vi "Get_Stat_Dots&Single_Frame_Displ-4.vi"(7 "Closing gaps":i32 min=1, 8 "[IN] error":errorcluster, 9 "[IN] Movie Values":T2 {"Particle Fil Setups"."Type of particle filter"."Measurement Parameter" items=["Center of Mass X", "Center of Mass Y", "First Pixel X", "First Pixel Y", "Bounding Rect Left", "Bounding Rect Top", "Bounding Rect Right", "Bounding Rect Bottom", "Max Feret Diameter Start X", "Max Feret Diameter Start Y", "Max Feret Diameter End X", "Max Feret Diameter End Y", "Max Horiz. Segment Length Left", "Max Horiz. Segment Length Right", "Max Horiz. Segment Length Row", "-", "Bounding Rect Width", "Bounding Rect Height", "Bounding Rect Diagonal", "Perimeter", "Convex Hull Perimeter", "Holes' Perimeter", "Max Feret Diameter", "Equivalent Ellipse Major Axis", "Equivalent Ellipse Minor Axis", "Equivalent Ellipse Minor Axis (Feret)", "Equivalent Rect Long Side", "Equivalent Rect Short Side", "Equivalent Rect Diagonal", "Equivalent Rect Short Side (Feret)", "Average Horiz. Segment Length", "Average Vert. Segment Length", "Hydraulic Radius", "Waddel Disk Diameter", "-", "Area", "Holes' Area", "Particle & Holes' Area", "Convex Hull Area", "Image Area", "-", "Number of Holes", "Number of Horiz. Segments", "Number of Vert. Segments", "-", "Orientation", "Max Feret Diameter Orientation", "-", "% Area/Image Area", "% Area/(Particle & Holes' Area)", "Ratio of Equivalent Ellipse Axes", "Ratio of Equivalent Rect Sides", "-", "Elongation Factor", "Compactness Factor", "Heywood Circularity Factor", "Type Factor", "-", "Sum X", "Sum Y", "Sum XX", "Sum XY", "Sum YY", "Sum XXX", "Sum XXY", "Sum XYY", "Sum YYY", "-", "Moment of Inertia XX", "Moment of Inertia XY", "Moment of Inertia YY", "Moment of Inertia XXX", "Moment of Inertia XXY", "Moment of Inertia XYY", "Moment of Inertia YYY", "Norm. Moment of Inertia XX", "Norm. Moment of Inertia XY", "Norm. Moment of Inertia YY", "Norm. Moment of Inertia XXX", "Norm. Moment of Inertia XXY", "Norm. Moment of Inertia XYY", "Norm. Moment of Inertia YYY", "Hu Moment 1", "Hu Moment 2", "Hu Moment 3", "Hu Moment 4", "Hu Moment 5", "Hu Moment 6", "Hu Moment 7"]}, 10 "dR max":dbl, 11 "dR min":dbl) -> (0 "error OUT":errorcluster, 1 "[OUT] Stationary Dots":T3(array[cluster]), 2 "[OUT] Displacements \nwith Length >1 Frame":dbl[][](array[numeric]), 3 "[OUT] (X,Y) Poten-\ntially Moving":dbl[][](array[numeric]), 5 "[OUT] Dot matrix after using \nsome filters which contains \ndots with increased statuses":i16[][](array[numeric]), 6 "[OUT] Unmoving\nsequences in array\nof frames":dbl[][](array[numeric]))   [LabVIEW 2013]
doc: "Top-level subVI for:\n1) calculation of initial displacements (with min and max displacement values)\n2) searching for unmoving particles and saving them in cluster / array\n3) highlighting the potentially unmoving particles"
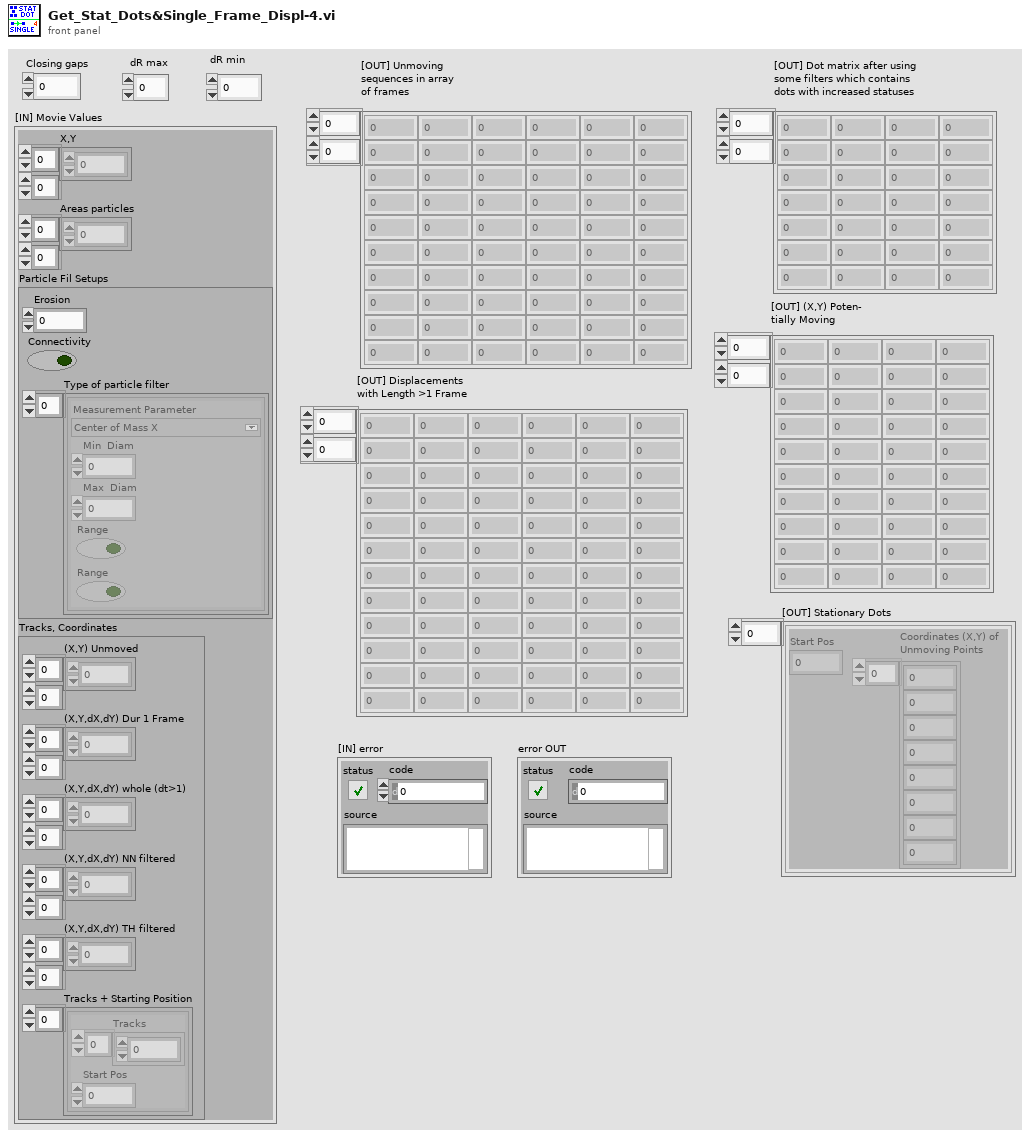
[diagram p1: front panel]
types:
  T1 = typedef "Particle Parameters" = i32
  T2 = cluster{"X,Y":dbl[][], "Areas particles":dbl[][], "Particle Fil Setups":cluster{"Erosion":i32, "Connectivity ":bool, "Type of particle filter":cluster{"Measurement Parameter":T1, "Min  Diam":dbl, "Max  Diam":dbl, "Range":bool, "Range":bool}[]}, "Tracks, Coordinates":cluster{"(X,Y) Unmoved":dbl[][], "(X,Y,dX,dY) Dur 1 Frame":dbl[][], "(X,Y,dX,dY) whole (dt>1)":dbl[][], "(X,Y,dX,dY) NN filtered":dbl[][], "(X,Y,dX,dY) TH filtered":dbl[][], "Tracks + Starting Position":cluster{"Tracks":dbl[], "Start Pos":i32}[]}}
  T3 = cluster{"Coordinates (X,Y) of\nUnmoving Points":dbl[], "Start Pos":i32}[]
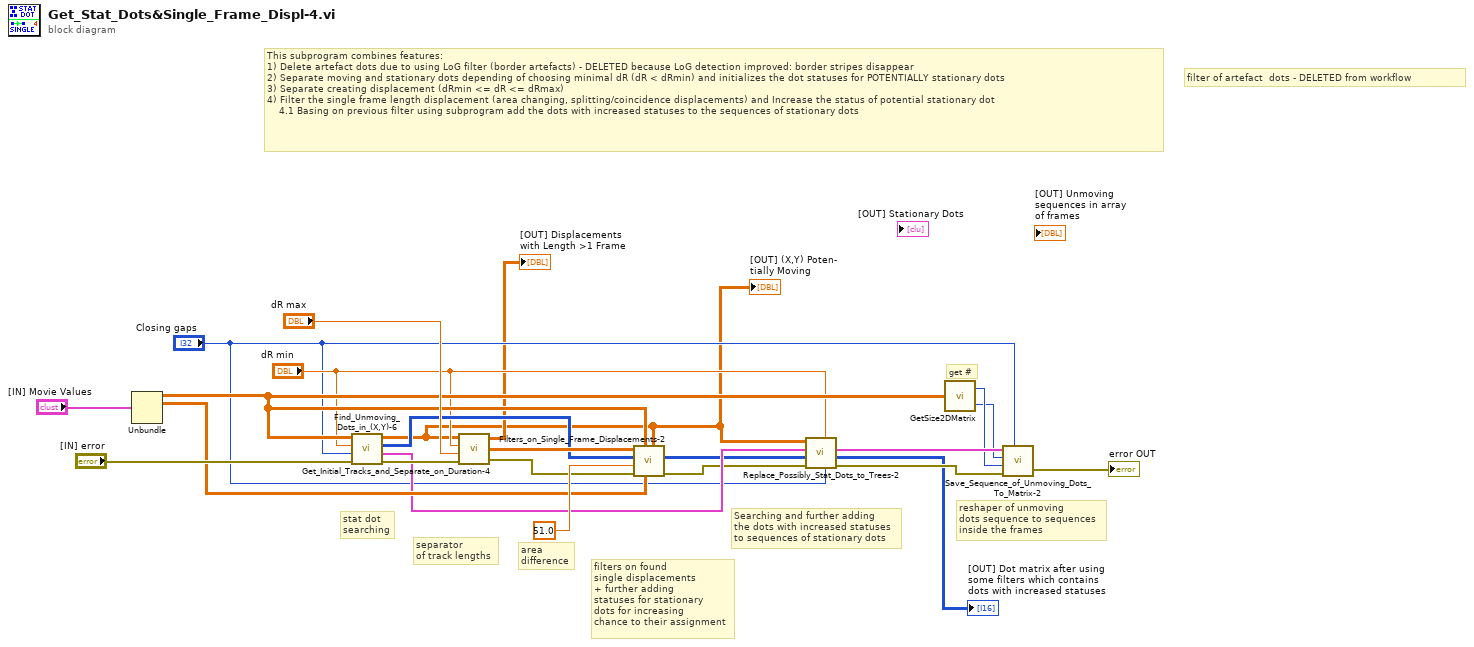
[diagram p0: block diagram]
diagram:
  # "Searching and further adding\nthe dots with increased statuses\nto sequences of stationary dots"
  # "This subprogram combines features:\n1) Delete artefact dots due to using LoG filter (border artefacts) - DELETED because LoG detection improved: border stripes disappear\n2) Separate moving and stationary dots depending of choosing minimal dR (dR < dRmin) and initializes the dot statuses for POTENTIALLY stationary dots\n3) Separate creating displacement (dRmin <= dR <= dRmax) \n4) Filter the single frame length displacement (area changing, splitting/coincidence displacements) and Increase the status of potential stationary dot\n    4.1 Basing on previous filter using subprogram add the dots with increased statuses to the sequences of stationary dots"
  # "filters on found \nsingle displacements\n+ further adding\nstatuses for stationary\ndots for increasing \nchance to their assignment"
  # "separator\nof track lengths"
  # "area \ndifference"
  # "reshaper of unmoving\ndots sequence to sequences\ninside the frames"
  # "stat dot\nsearching"
  # "filter of artefact  dots - DELETED from workflow"
  # "get #"
  n1 = Unbundle("[IN] Movie Values") -> ("X,Y"=w17:dbl[][], "Areas particles"=w15:dbl[][])  [unwired: 2 out]
  n2 = call "Find_Unmoving_Dots_in_(X,Y)-6.vi"("error IN"="[IN] error", "Gaps for closing"="Closing gaps", "dR min"="dR min", "[IN] Primary (X,Y)"=w17) -> ("error OUT"=w21:errorcluster, "[OUT] Stationary Dots"=w14:T3, "[OUT] Dot matrix\nwith statuses for\nmoving and poten-\ntially moving dots"=w19:i16[][], "[OUT] (X,Y) Potentially Moving"=w4:dbl[][])
  "[OUT] (X,Y) Poten-\ntially Moving" <- w4
  n3 = call "Get_Initial_Tracks_and_Separate_on_Duration-4.vi"("error IN"=w21, "dR max"="dR max", "dR min"="dR min", "[IN] Potential\nMoving Dots (X,Y)"=w4) -> ("error OUT"=w16:errorcluster, "Displacements =1 Frame"=w20:dbl[][], "Displacements >1 Frame"=→"[OUT] Displacements \nwith Length >1 Frame":dbl[][])
  n4 = call "Filters_on_Single_Frame_Displacements-2.vi"("[IN] Possibly\nMoving (X,Y)"=w4, "Areas of\nobjects"=w15, "[IN] Primary \nCoordinates (X,Y)"=w17, "error IN"=w16, "% DIfference between \nParticle Squares"=51.0 ("% DIfference between \nParticle Squares"), "[IN] Dot matrix with \nstatuses for  potentially \nmoving dots"=w19, "[IN] Potential\ndisplacement \n(X,Y,dX,dY)"=w20) -> ("error OUT"=w12:errorcluster, "[OUT] Dot matrix with \nstatuses for potentially \nmoving dots"=w13:i16[][])  [unwired: 2 in, 1 out]
  n5 = call "Replace_Possibly_Stat_Dots_to_Trees-2.vi"("[IN] Possibly\nMoving (X,Y)"=w4, "[IN] Stationary Dots"=w14, "[IN] Dot matrix after using \nsome filters which contains \ndots with increased statuses"=w13, "error IN"=w12, "[IN] dR min"="dR min", "Closing gaps"="Closing gaps") -> ("[OUT] Stationary Dots"=w10:T3, "[OUT] Dot matrix after using \nsome filters which contains \ndots with increased statuses"=→"[OUT] Dot matrix after using \nsome filters which contains \ndots with increased statuses":i16[][], "error OUT"=w9:errorcluster)  [unwired: 1 in]
  n6 = call "GetSize2DMatrix.vi"("Array IN (2D)"=w17) -> ("# Cols"=w7:i32, "# Rows"=w6:i32)
  n7 = call "Save_Sequence_of_Unmoving_Dots_To_Matrix-2.vi"("[IN] Stationary Dots"=w10, "# rows"=w6, "# cols"=w7, "error IN"=w9, "[IN] # Gaps"="Closing gaps") -> ("error OUT"=→"error OUT":errorcluster)  [unwired: 1 out]
